vi "Set pts at min.vi"(11 "Waveform parameters":T1 {"StartCurrent" min=0.001}) -> (3 "Waveform parameters out":T1={"StartCurrent"=1.0, "MaximumCurrent (mA)"=3.0, "Number oif pulses"=3, "Ramp length"=20, "Top length"=4, "Exponent"=1, "CurrentStep "=1.0, "Baseline length"=8, "Next current step"=0.0} {"StartCurrent" min=0.001})   [LabVIEW 2015]
uses:
  Original Waveform parameters.ctl
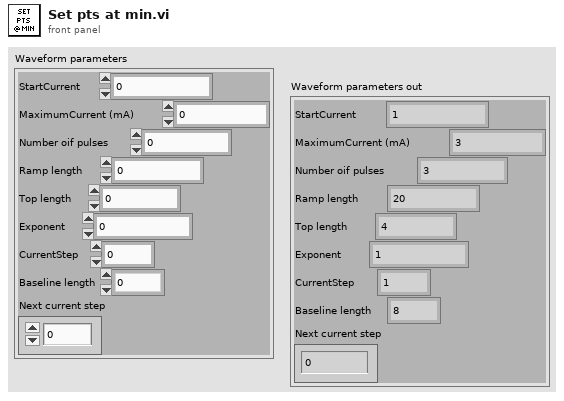
[diagram p1: front panel]
types:
  T1 = typedef "Original Waveform parameters.ctl" = cluster{"StartCurrent":dbl, "MaximumCurrent (mA)":dbl, "Number oif pulses":i32, "Ramp length":i32, "Top length":i32, "Exponent":i16, "CurrentStep ":dbl, "Baseline length":i32, "Next current step":dbl}
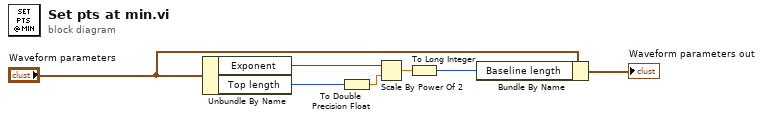
[diagram p0: block diagram]
diagram:
  n1 = Unbundle By Name("Waveform parameters") -> ("Exponent"=w6:i16, "Top length"=w5:i32)
  n2 = To Double Precision Float(number=w5) -> (double precision float=w4:dbl)
  n3 = Scale By Power Of 2(n=w6, x=w4) -> (x*2^n=w3:dbl)
  n4 = To Long Integer(number=w3) -> (32bit integer=w1:i32)
  n5 = Bundle By Name(cluster="Waveform parameters", "Baseline length"=w1) -> (→"Waveform parameters out":T1)
